vi "Save Hotkey.vi"(7 "Hotkey Type":T1, 8 "error in (no error)":errorcluster, 10 "Hotkey":T2(array[ring]), 11 "File Path":path) -> (0 "error out":errorcluster)   [LabVIEW 2020, in "MacroAssert.lvlib"]
doc: "Saves <B>Hotkey</B> and its associated <B>Hotkey Type</B> to a config file."
uses:
  MacroAssert.lvlib
  <vilib>/Utility/config.llb/NI_LVConfig.lvlib
  <vilib>/Utility/config.llb/Write Key (String).vi
  CTLs/Hotkey Type.ctl
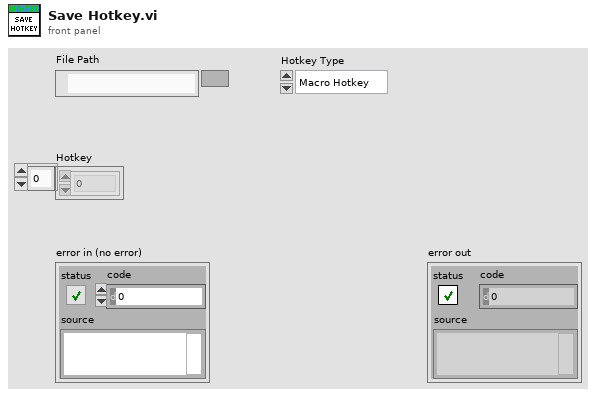
[diagram p1: front panel]
types:
  T1 = typedef "MacroAssert.lvlib/Hotkey Type.ctl" = enum16{"Macro Hotkey", "Abort Hotkey"}
  T2 = enum16{"0", "1", "2", "3", "4", "5", "6", "7", "8", "9", "A", "B", "C", "D", "E", "F", "G", "H", "I", "J", "K", "L", "M", "N", "O", "P", "Q", "R", "S", "T", "U", "V", "W", "X", "Y", "Z", "F1", "F2", "F3", "F4", "F5", "F6", "F7", "F8", "F9", "F10", "F11", "F12", "F13", "F14", "F15", "ADD", "BACK", "BACKSLASH", "CAPITAL", "COMMA", "DECIMAL", "DELETE", "DIVIDE", "DOWN", "END", "EQUALS", "ESCAPE", "GRAVE (`)", "HOME", "INSERT", "LBRACKET", "LCONTROL", "LEFT", "L ALT", "LSHIFT", "LWIN", "MINUS", "MULTIPLY", "NEXT", "NUMLOCK", "NUMPAD_0", "NUMPAD_1", "NUMPAD_2", "NUMPAD_3", "NUMPAD_4", "NUMPAD_5", "NUMPAD_6", "NUMPAD_7", "NUMPAD_8", "NUMPAD_9", "PAUSE", "PERIOD", "PRIOR (PG UP)", "RBRACKET", "RCONTROL", "RETURN", "RIGHT", "R ALT", "RSHIFT", "RWIN", "SCROLL", "SEMICOLON", "SLASH", "SPACE", "SUBTRACT", "TAB", "UP", "ENTER (num pad)", "' (quote)"}[]
  T3 = typedef "NI_LVConfig.lvlib/Config Data RefNum.ctl" = refnum<k1>
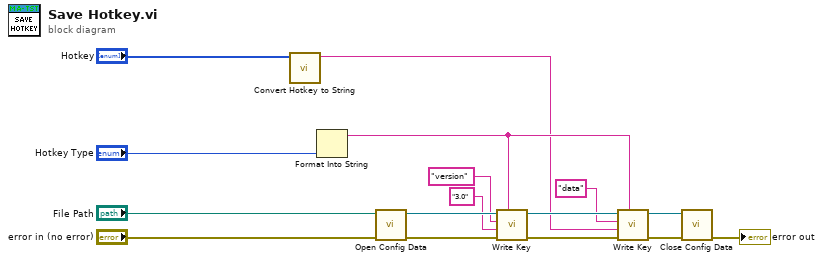
[diagram p0: block diagram]
diagram:
  n1 = call "Convert Hotkey to String.vi"("Hotkey"="Hotkey") -> ("String"=w1:string)  [unwired: 10 in]
  n2 = Format Into String("Hotkey Type") -> (resulting string=w8:string)  [unwired: 3 in, 1 out]
  n3 = call <vilib>:"Open Config Data.vi"("error in (no error)"="error in (no error)", "configuration file path"="File Path") -> ("error out"=w10:errorcluster, "refnum"=w15:T3)  [unwired: 7 in, 1 out]
  n4 = call-poly <vilib>:"Write Key.vi"("section"=w8, "error in (no error)"=w10, "value"="3.0" ("key"), "key"="version", "refnum"=w15) -> ("error out"=w9:errorcluster, "refnum out"=w16:T3)  [unwired: 4 in, 1 out]
  n5 = call-poly <vilib>:"Write Key.vi"("section"=w8, "error in (no error)"=w9, "value"=w1, "key"="data", "refnum"=w16) -> ("error out"=w14:errorcluster, "refnum out"=w13:T3)  [unwired: 4 in, 1 out]
  n6 = call <vilib>:"Close Config Data.vi"("error in (no error)"=w14, "refnum"=w13) -> ("error out"=→"error out":errorcluster)  [unwired: 8 in, 1 out]
